vi "InputClk_Status.vi"(0 "COMPORT":refnum<visa-resource-name>="COM6", 11 "error in (no error)":errorcluster, 12 "CLK_USAGE":u16(ring) items=["EXT CLK", "INT CLK"], 13 "Open Serial":bool, 14 "Close Serial":bool) -> (3 "PllSuccess?(T)":bool, 15 "error out":errorcluster)   [LabVIEW 2018]
panel:
  out "count?(t)":bool
  out "result(i32)":i32
  out "Reg 0x06":string
  out "Readback Success?(t)":bool
  # "THIS VI IS DESIGNED TO DETECT THE PRESENCE OF EXTERNAL CLOCK\nPRESENCE AT THE SiTime IN_0.\nSelect \"CLK_USAGE\" def = EXT CLK\nIF Readback  = 0 \n OR \nIF CLK_USAGE = INT CLK AND Readback = 44\nTHEN PllSuccess = TRUE\nELSE = FLAG Operator to check cables\nUser has 3 tries or option to end without success"
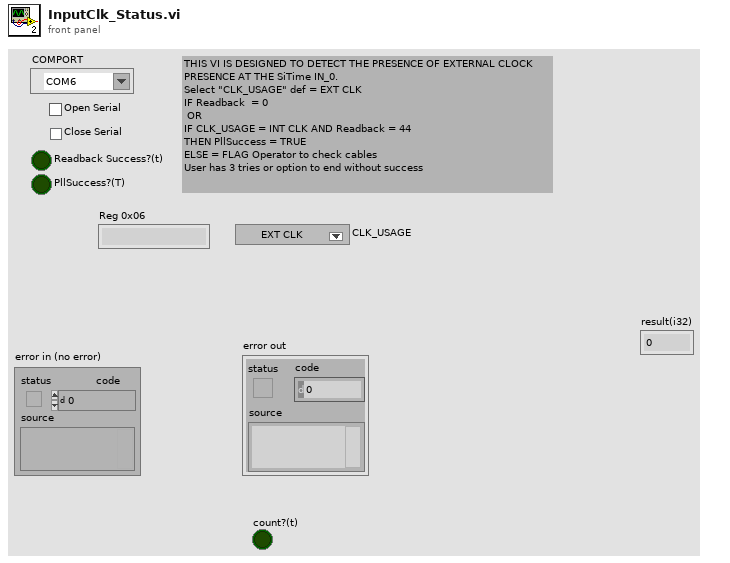
[diagram p1: front panel]
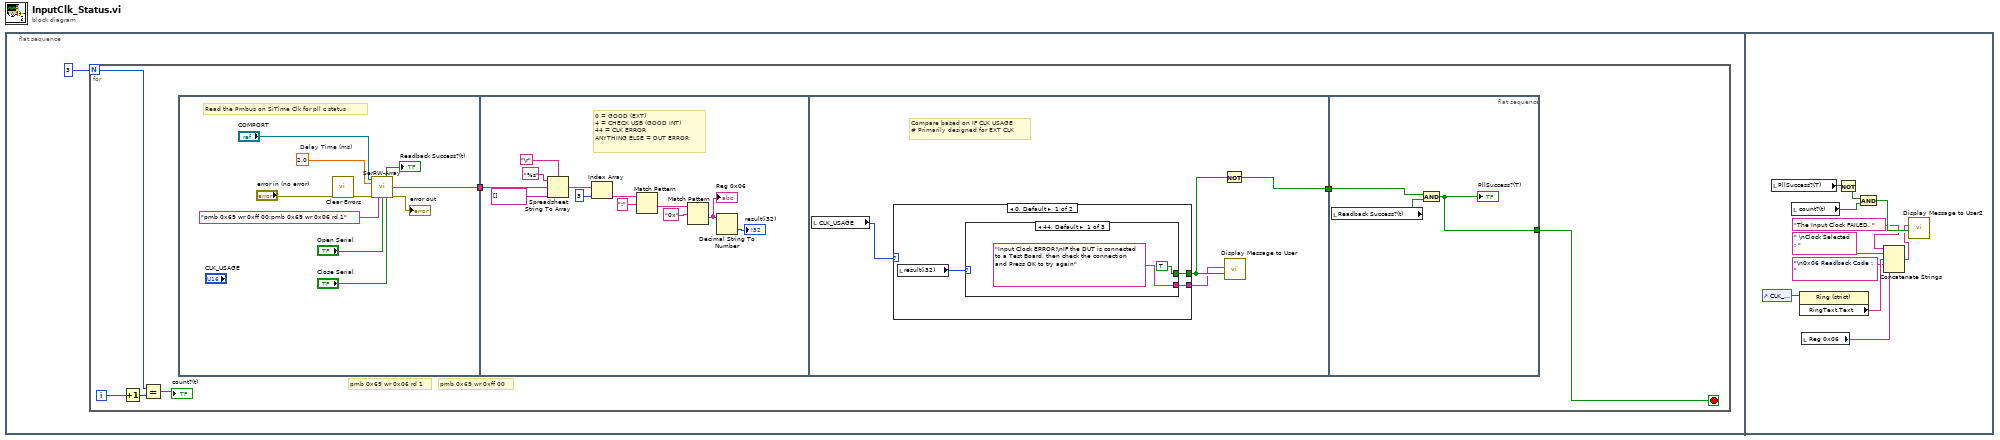
[diagram p0: block diagram]
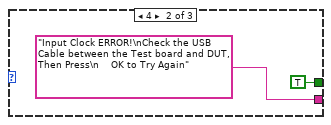
[diagram p2: hidden frame]
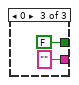
[diagram p3: hidden frame]
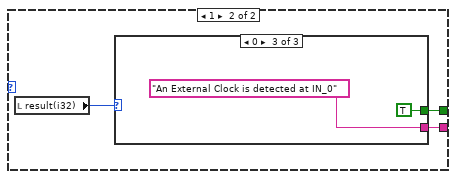
[diagram p4: hidden frame]
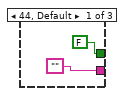
[diagram p5: hidden frame]
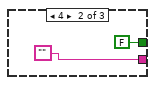
[diagram p6: hidden frame]
diagram:
  n1 = flat-sequence {
    frame #0 {
      n2 = for {
        N: 3 -> [w5]
        i -> [w4]
        stop <- w6 stop-if-true
        # "pmb 0x69 wr 0xff 00"
        # "pmb 0x69 wr 0x06 rd 1"
        n3 = Increment(x=w4) -> (x+1=w3:i32)
        n4 = Equal?(x=w5, y=w3) -> (x = y?=→"count?(t)":bool)
        n5 = flat-sequence {
          tunnel: [w13] -> w8
          tunnel: w8 -> [w21]
          tunnel: [w31] -> w7
          tunnel: w7 -> [w54]
          tunnel: [w53] -> w6
          frame #0 {
            w10 = 2.0  # Delay Time (ms)
            # "Read the Pmbus on SiTime Clk for pll c status"
            n6 = call <vilib>:"Clear Errors.vi"("error in (no error)"="error in (no error)") -> ("error out"=w11:errorcluster)  [unwired: 5 in, 1 out]
            n7 = call "SerRW-Array.vi"("COMPORT"="COMPORT", "Delay Time (ms)"=w10, "error in (no error)"=w11, "Command ( ; seperation)"="pmb 0x69 wr 0xff 00;pmb 0x69 wr 0x06 rd 1", "Open Serial"="Open Serial", "Close Serial"="Close Serial") -> ("All Success"=→"Readback Success?(t)":bool, "string"=w13:string, "error out"=→"error out":errorcluster)  [unwired: 3 in, 4 out]
          }
          frame #1 {
            # "0 = GOOD (EXT)\n4 = CHECK USB (GOOD INT)\n44 = CLK ERROR\nANYTHING ELSE = DUT ERROR"
            n8 = Spreadsheet String To Array(delimiter (Tab)="\r", format string="%s", spreadsheet string=w21, array type (2D Dbl)=string[] []) -> (array=w26:string[])
            n9 = Index Array(array=w26, index=3) -> (element=w27:string)
            n10 = Match Pattern(string=w27, regular expression=":") -> (after substring=w28:string)  [unwired: 1 in, 3 out]
            n11 = Match Pattern(string=w28, regular expression="0x") -> (after substring=w29:string)  [unwired: 1 in, 3 out]
            "Reg 0x06" <- w29
            n12 = Decimal String To Number(string=w29) -> (number=→"result(i32)":i32)  [unwired: 2 in, 1 out]
          }
          frame #2 {
            # "Compare based on IF CLK USAGE\n# Primarily designed for EXT CLK"
            n13 = local read "CLK_USAGE"() -> (w32:u16)
            n14 = case shown="0, Default" w32 {
              tunnel: [w36 w45] -> w34
              tunnel: [w35 w44] -> w33
              frame 0, Default {
                n15 = local read "result(i32)"() -> (w37:i32)
                n16 = case shown="44, Default" w37 {
                  tunnel: [TRUE ("Enable") TRUE ("Enable") FALSE ("Enable")] -> w36
                  tunnel: ["Input Clock ERROR!\nIF the DUT is connected to a Test Board, then check the connection and Press OK to try again" "Input Clock ERROR!\nCheck the USB Cable between the Test board and DUT, Then Press\n    OK to Try Again" ""] -> w35
                  frame 44, Default {
                  }
                  frame 4 {
                  }
                  frame 0 {
                  }
                }
              }
              frame 1 {
                n17 = local read "result(i32)"() -> (w46:i32)
                n18 = case shown="0" w46 {
                  tunnel: [FALSE ("Enable") FALSE ("Enable") TRUE ("Enable")] -> w45
                  tunnel: ["" "" "An External Clock is detected at IN_0"] -> w44
                  frame 44, Default {
                  }
                  frame 4 {
                  }
                  frame 0 {
                  }
                }
              }
            }
            n19 = Not(x=w34) -> (.not. x?=w31:bool)
            n20 = call "Display Message to User"("Enable"=w34, "Message"=w33) -> ()  [unwired: 8 in, 2 out]
          }
          frame #3 {
            n21 = local read "Readback Success?(t)"() -> (w55:bool)
            n22 = And(x=w54, y=w55) -> (x .and. y?=w53:bool)
            "PllSuccess?(T)" <- w53
          }
        }
      }
    }
    frame #1 {
      n23 = control-ref of="CLK_USAGE"() -> (w58:refnum<vi>)
      n24 = local read "PllSuccess?(T)"() -> (w66:bool)
      n25 = local read "count?(t)"() -> (w64:bool)
      n26 = property class="Ring (strict)"(reference=w58) -> ("RingText.Text"=w61:string)  [unwired: 1 in, 2 out]
      n27 = local read "Reg 0x06"() -> (w56:string)
      n28 = Not(x=w66) -> (.not. x?=w65:bool)
      n29 = And(x=w65, y=w64) -> (x .and. y?=w63:bool)
      n30 = Concatenate Strings("The Input Clock FAILED. " ("Message"), " \nClock Selected : " ("Message"), w61, "\n0x06 Readback Code : " ("string"), w56) -> (w59:string)
      n31 = call "Display Message to User2"("Enable"=w63, "Message"=w59) -> ()  [unwired: 8 in, 2 out]
    }
  }
